vi "TimeDateToSQLDateTime.vi"(10 "TimeDate":string) -> (0 "time stamp":timestamp, 1 "StartMDY":string, 2 "date/timeSQL":string)   [LabVIEW 2012]
uses:
  <vilib>/Utility/miscctls.llb/LVDateTimeRec.ctl
panel:
  in  "date time rec":T1
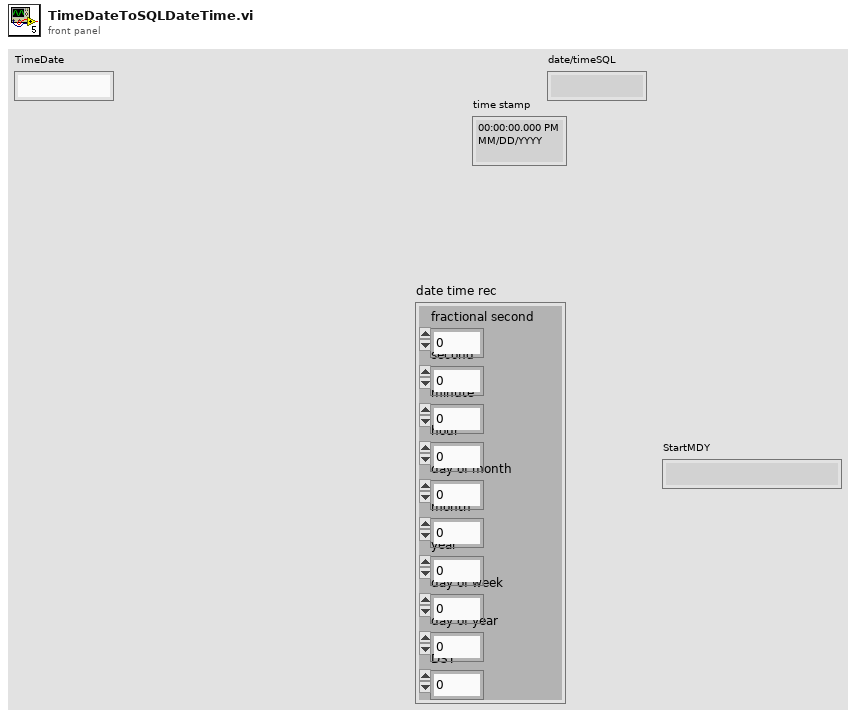
[diagram p1: front panel]
types:
  T1 = typedef "LVDateTimeRec.ctl" = cluster{"fractional second":dbl, "second":i32, "minute":i32, "hour":i32, "day of month":i32, "month":i32, "year":i32, "day of week":i32, "day of year":i32, "DST":i32}
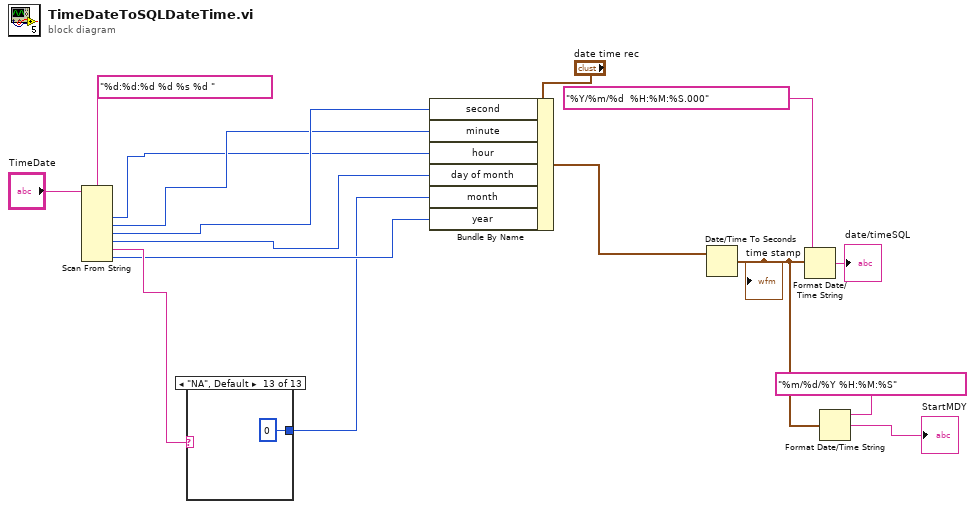
[diagram p0: block diagram]
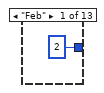
[diagram p2: hidden frame]
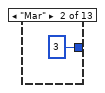
[diagram p3: hidden frame]
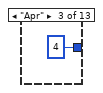
[diagram p4: hidden frame]
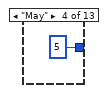
[diagram p5: hidden frame]
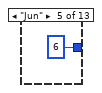
[diagram p6: hidden frame]
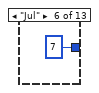
[diagram p7: hidden frame]
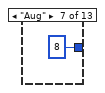
[diagram p8: hidden frame]
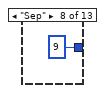
[diagram p9: hidden frame]
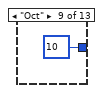
[diagram p10: hidden frame]
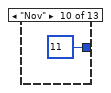
[diagram p11: hidden frame]
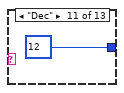
[diagram p12: hidden frame]
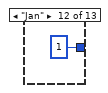
[diagram p13: hidden frame]
diagram:
  n1 = Scan From String(format string="%d:%d:%d %d %s %d ", input string="TimeDate") -> (output 1=w8:i32, output 2=w9:i32, output 3=w10:i32, output 4=w11:i32, output 5=w15:string, output 6=w13:i32)  [unwired: 8 in, 3 out]
  n2 = case shown="\"NA\", Default" w15 {
    tunnel: [2 3 4 5 6 7 8 9 10 11 12 1 0] -> w12
    frame "Feb" {
    }
    frame "Mar" {
    }
    frame "Apr" {
    }
    frame "May" {
    }
    frame "Jun" {
    }
    frame "Jul" {
    }
    frame "Aug" {
    }
    frame "Sep" {
    }
    frame "Oct" {
    }
    frame "Nov" {
    }
    frame "Dec" {
    }
    frame "Jan" {
    }
    frame "NA", Default {
    }
  }
  n3 = Bundle By Name(cluster="date time rec", "second"=w10, "minute"=w9, "hour"=w8, "day of month"=w11, "month"=w12, "year"=w13) -> (w5:T1)
  n4 = Date/Time To Seconds(2:w5) -> (0:w1:timestamp)  [unwired: 1 in]
  "time stamp" <- w1
  n5 = Format Date/Time String(time format string (%c)="%Y/%m/%d  %H:%M:%S.000", seconds (now)=w1) -> (date/time string=→"date/timeSQL":string)  [unwired: 1 in]
  n6 = Format Date/Time String(time format string (%c)="%m/%d/%Y %H:%M:%S", seconds (now)=w1) -> (date/time string=→"StartMDY":string)  [unwired: 1 in]
